vi "GetOldest__slk_tc.vi"(0 "tree control in":refnum<class "TreeControl.lvclass">, 11 "error in (no error)":errorcluster) -> (4 "tree control out":refnum<class "TreeControl.lvclass">, 6 "oldest children tags":string[](array[string]), 15 "error out":errorcluster)   [LabVIEW 2020, in "TreeControl.lvclass"]
doc: "Collects and returns all tags of oldest (leftmost) items in the tree."
uses:
  Library/TreeControl.lvclass
  Library/TreeControl.lvclass/TreeControl.ctl
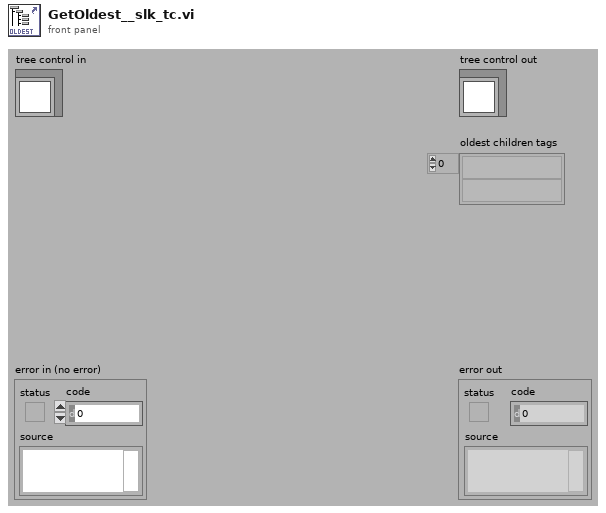
[diagram p1: front panel]
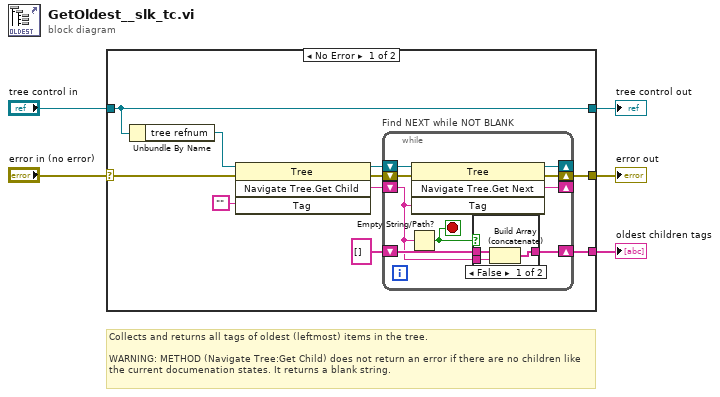
[diagram p0: block diagram]
diagram:
  # "Collects and returns all tags of oldest (leftmost) items in the tree.\n\nWARNING: METHOD (Navigate Tree:Get Child) does not return an error if there are no children like the current documenation states. It returns a blank string."
  n1 = case shown="No Error" "error in (no error)" {
    selector: "error in (no error)" -> [w11 w30]
    tunnel: [w10 w30] -> w4
    tunnel: [w8 w29] -> w2
    tunnel: "tree control in" -> [w8 w29]
    tunnel: [w6 _] -> w1
    frame No Error {
      n2 = Unbundle By Name(w8) -> ("tree refnum"=w7:refnum<vi>)
      n3 = invoke class="Tree" method="Navigate Tree.Get Child"(reference=w7, error in=w11, "Tag"="") -> (reference out=w14:refnum<vi>, error out=w15:errorcluster, "Navigate Tree:Get Child"=w13:string)  [unwired: 1 in, 1 out]
      n4 = while "Find NEXT while NOT BLANK" {
        shift-right: [w21] -> w10
        shift-left: w15 -> [w23]
        shift-right: [w22] -> _
        shift-left: w14 -> [w24]
        shift-right: [w20] -> _
        shift-left: w13 -> [w17]
        shift-right: [w18] -> w6
        shift-left: string[] [] -> [w19]
        stop <- w16 stop-if-true
        n5 = Empty String/Path?(string/path=w17) -> (empty?=w16:bool)
        n6 = invoke class="Tree" method="Navigate Tree.Get Next"(reference=w24, error in=w23, "Tag"=w17) -> (reference out=w22:refnum<vi>, error out=w21:errorcluster, "Navigate Tree:Get Next Item"=w20:string)  [unwired: 1 in, 1 out]
        n7 = case shown="False" w16 {
          tunnel: w19 -> [w27 w28]
          tunnel: [w26 w28] -> w18
          tunnel: w17 -> [w25 _]
          frame False {
            n8 = Build Array (concatenate)(w27, w25) -> (w26:string[])
          }
          frame True {
          }
        }
      }
    }
    frame Error {
    }
  }
  "error out" <- w4
  "tree control out" <- w2
  "oldest children tags" <- w1
